vi "Angular Speed.vi"(4 "error in (no error)":errorcluster, 5 "avg on n pulses (1:no average)":i32=1, 6 "pulse/revolution (1)":dbl=1.0 format="%.2f", 7 "pulse positions [s]":dbl[](array[numeric]) format="%.2f") -> (0 "error out":errorcluster, 3 "speed profile":T1 {"speed [RPM]" format="%.2f"; "time [s]" format="%.2f"})   [LabVIEW 2017]
doc: "Computes the angular speed at each pulse edge contained in <B>pulse positions [s]</B>."
uses:
  <vilib>/addons/Sound and Vibration/Order Analysis/Tach Process/SubVIs/speed profile.ctl
  <vilib>/addons/Sound and Vibration/Order Analysis/Tach Process/SoundVib_TachProcess.lvlib
panel:
  in  "reset? (True)":bool=TRUE
  # "Angular Speed (at edges)"
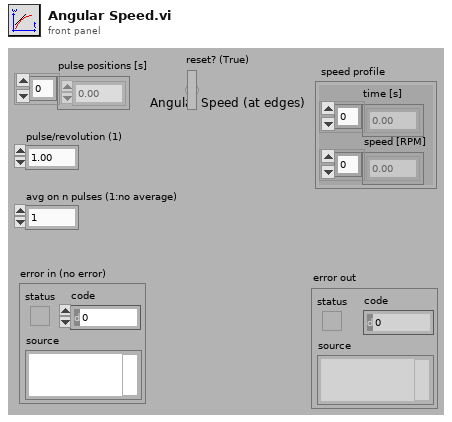
[diagram p1: front panel]
types:
  T1 = typedef "SoundVib_TachProcess.lvlib/speed profile.ctl" = cluster{"time [s]":dbl[], "speed [RPM]":dbl[]}
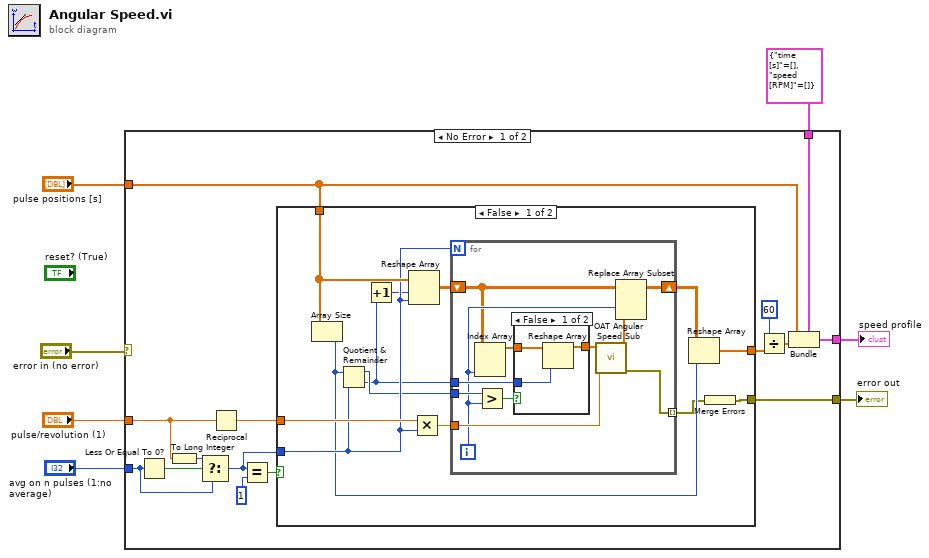
[diagram p0: block diagram]
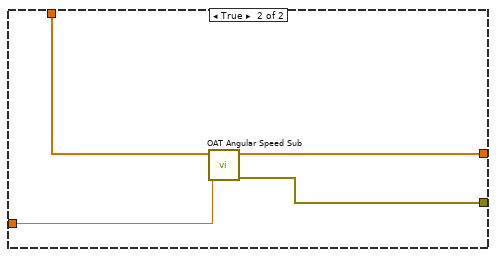
[diagram p3: hidden frame]
diagram:
  n1 = case shown="No Error" "error in (no error)" {
    selector: "error in (no error)" -> [_ w55]
    tunnel: "avg on n pulses (1:no average)" -> [w21 _]
    tunnel: "pulse positions [s]" -> [w14 _]
    tunnel: [w13 w56] -> w5
    tunnel: "pulse/revolution (1)" -> [w10 _]
    tunnel: [w9 w55] -> w3
    tunnel: T1 {"time [s]"=[], "speed [RPM]"=[]} ("speed profile") -> [w8 w56]
    frame No Error {
      n2 = Less Or Equal To 0?(x=w21) -> (x <= 0?=w22:bool)
      n3 = To Long Integer(number=w10) -> (32bit integer=w15:i32)
      n4 = Select(t=w15, s=w22, f=w21) -> (s? t:f=w17:i32)
      n5 = Reciprocal(x=w10) -> (1/x=w18:dbl)
      n6 = Equal?(x=w17, y=1) -> (x = y?=w19:bool)
      n7 = case shown="False" w19 {
        tunnel: w14 -> [w35 w54]
        tunnel: w18 -> [w34 w53]
        tunnel: [w25 w52] -> w11
        tunnel: w17 -> [w33 _]
        tunnel: [w23 w51] -> w9
        frame False {
          n8 = Array Size(array=w35) -> (size(s)=w31:i32)
          n9 = Quotient & Remainder(x=w31, y=w33) -> (x-y*floor(x/y)=w30:i32, floor(x/y)=w28:i32)
          n10 = Increment(x=w28) -> (x+1=w29:i32)
          n11 = Reshape Array(w35, w29, w33) -> (w27:dbl[][])
          n12 = Multiply(x=w34, y=w33) -> (x*y=w32:dbl)
          n13 = for {
            N: w33 -> [_]
            tunnel: w32 -> [w45]
            tunnel: w30 -> [w43]
            tunnel: w28 -> [w41]
            shift-right: [w37] -> w26
            shift-left: w27 -> [w38]
            tunnel: [w36] -> w24 mode=indexing
            i -> [w40]
            n14 = Index Array(array=w38, index (col)=w40) -> (element=w46:dbl[])  [unwired: 1 in]
            n15 = Greater?(x=w43, y=w40) -> (0:w42:bool)
            n16 = case shown="False" w42 {
              tunnel: w46 -> [w49 w50]
              tunnel: [w48 w50] -> w44
              tunnel: w41 -> [w47 _]
              frame False {
                n17 = Reshape Array(w49, w47) -> (w48:dbl[])
              }
              frame True {
              }
            }
            n18 = call <vilib>:"OAT Angular Speed Sub.vi"("deltaX"=w45, "Y[n]"=w44) -> ("error out"=w36:errorcluster, "dY/dX[n]"=w39:dbl[])  [unwired: 8 in]
            n19 = Replace Array Subset(array=w38, new element=w39, index (col)=w40) -> (w37:dbl[][])  [unwired: 1 in]
          }
          n20 = Reshape Array(w26, w31) -> (w25:dbl[])
          n21 = Merge Errors(w24) -> (w23:errorcluster)
        }
        frame True {
          n22 = call <vilib>:"OAT Angular Speed Sub.vi"("deltaX"=w53, "Y[n]"=w54) -> ("error out"=w51:errorcluster, "dY/dX[n]"=w52:dbl[])  [unwired: 8 in]
        }
      }
      n23 = Divide(x=60, y=w11) -> (x/y=w12:dbl[])
      n24 = Bundle(cluster=w8, "time [s]"=w14, "speed [RPM]"=w12) -> (w13:T1)
    }
    frame Error {
    }
  }
  "speed profile" <- w5
  "error out" <- w3
